vi "tls http parse header.vi"(7 "lvlibretls connection in":refnum<class "lvlibretls connection.lvclass">, 10 "data in":string, 11 "application request":T1) -> (2 "abort":bool, 3 "application request out":T1)   [LabVIEW 2016, in "Basic HTTPS server.lvclass"]
uses:
  Basic HTTPS server.lvclass
  http request.ctl
  http method.ctl
  HTTP headers/http header data.ctl
  lvlibtls/socket connection/lvlibretls connection.lvclass
  <vilib>/dlg_ctls.llb/Space Constant.vi
  HTTP headers/http add header to set.vi
  HTTP headers/http headers.lvlib
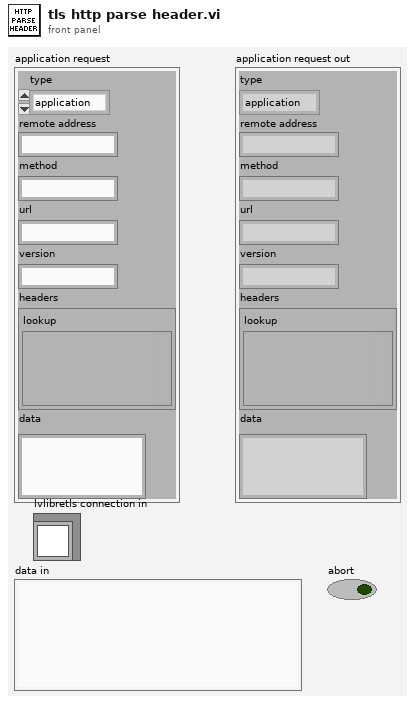
[diagram p1: front panel]
types:
  T1 = typedef "Basic HTTPS server.lvclass/http request.ctl" = cluster{"type":T2, "remote address":string, "method":string, "url":string, "version":string, "headers":T3, "data":string}
  T2 = typedef "Basic HTTPS server.lvclass/http method.ctl" = enum16{"application", "error", "upgrade"}
  T3 = typedef "http headers.lvlib/http header data.ctl" = cluster{"lookup":variant}
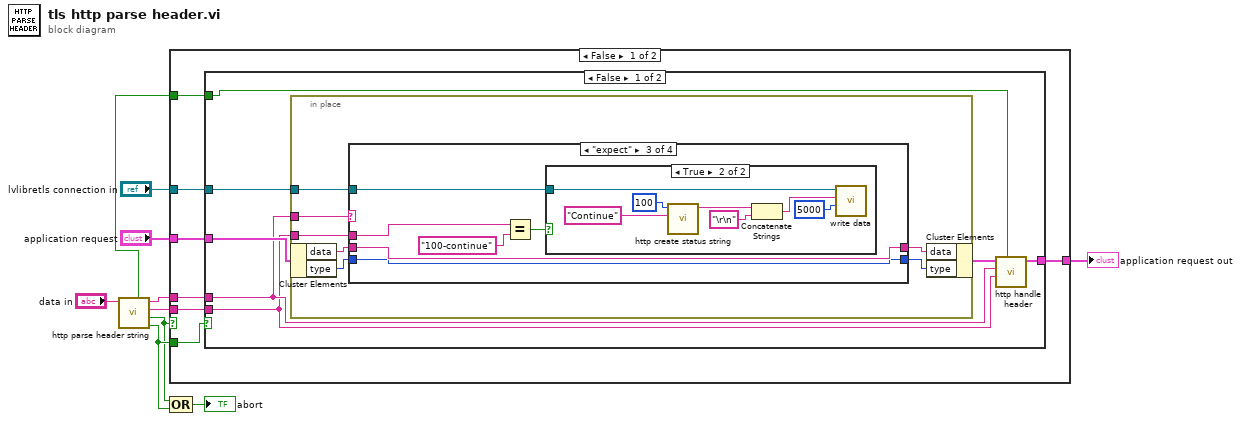
[diagram p0: block diagram]
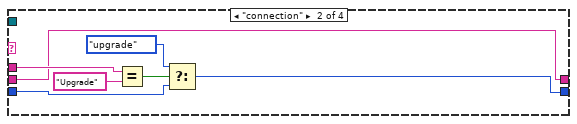
[diagram p3: hidden frame]
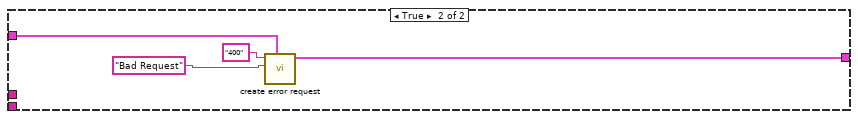
[diagram p6: hidden frame]
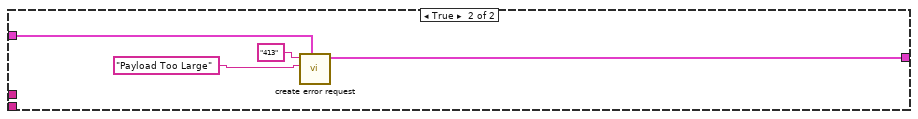
[diagram p7: hidden frame]
diagram:
  n1 = call "http parse header string.vi"("raw string"="data in") -> ("no field name"=w8:bool, "no crlf"=w7:bool, "header field data"=w3:string, "header field name"=w4:string, "continuation"=w6:bool)  [unwired: 6 in]
  n2 = case shown="False" w7 {
    tunnel: w8 -> [w17 _]
    tunnel: w6 -> [w16 _]
    tunnel: [w15 w60] -> w5
    tunnel: w4 -> [w14 _]
    tunnel: w3 -> [w13 _]
    tunnel: "application request" -> [w12 w61]
    tunnel: "lvlibretls connection in" -> [w11 _]
    frame False {
      n3 = case shown="False" w17 {
        tunnel: w16 -> [w24 _]
        tunnel: [w22 w56] -> w15
        tunnel: w14 -> [w20 _]
        tunnel: w13 -> [w19 _]
        tunnel: w12 -> [w21 w57]
        tunnel: w11 -> [w18 _]
        frame False {
          n4 = in-place {
            in-place-border: w20 -> [w31]
            in-place-border: w19 -> [w28]
            in-place-border: w18 -> [w25]
            n5 = in-place-cluster #1(w21) -> ("data"=w29:string, "type"=w26:T2)
            n6 = case shown="\"expect\"" w31 {
              selector: w31 -> [w33 _ _ _]
              tunnel: [w33 w34 w46 w55] -> w30
              tunnel: w29 -> [_ w34 w46 w55]
              tunnel: w28 -> [_ w39 w42 _]
              tunnel: [w32 w36 w45 w54] -> w27
              tunnel: w26 -> [w32 w35 w45 w54]
              tunnel: w25 -> [_ _ w41 _]
              frame "content-length", "transfer-encoding" {
              }
              frame "connection" {
                n7 = Equal?(x=w39, y="Upgrade" ("name")) -> (x = y?=w38:bool)
                n8 = Select(t=http_method."upgrade", s=w38, f=w35) -> (s? t:f=w36:T2)
              }
              frame "expect" {
                n9 = Equal?(x=w42, y="100-continue") -> (x = y?=w43:bool)
                n10 = case shown="True" w43 {
                  tunnel: w41 -> [_ w47]
                  frame False {
                  }
                  frame True {
                    n11 = call "http create status string.vi"("status string"="Continue", "reason code"=u16 100) -> ("status line"=w51:string)  [unwired: 9 in]
                    n12 = Concatenate Strings(w51, "\r\n" ("string")) -> (w48:string)
                    n13 = call "write data.vi"("timeout"=5000, "data"=w48, "lvlibretls connection in"=w47) -> ()  [unwired: 7 in, 2 out]
                  }
                }
              }
              frame Default {
              }
            }
            n14 = in-place-cluster #1("data"=w30, "type"=w27) -> (w23:T1)
          }
          n15 = call "http handle header.vi"("continuation"=w24, "header field data"=w19, "header field name"=w20, "application request in"=w23) -> ("application request out"=w22:T1)  [unwired: 7 in]
        }
        frame True {
          n16 = call "create error request.vi"("incoming request"=w57, "reason"="Bad Request" ("status string"), "code"="400") -> ("element"=w56:T1)  [unwired: 8 in]
        }
      }
    }
    frame True {
      n17 = call "create error request.vi"("incoming request"=w61, "reason"="Payload Too Large" ("status string"), "code"="413") -> ("element"=w60:T1)  [unwired: 8 in]
    }
  }
  "application request out" <- w5
  n18 = Compound Arithmetic op=OR(w7, w8) -> (→"abort":bool)
